vi "Cuboid Z test.vi"(1 "Cuboid 2":T1={"Vertices (x, y)"=[[0.0, 0.0], [0.0, 0.0], [0.0, 0.0], [0.0, 0.0]], "Zmin"=0.0, "Zmax"=0.0, "Centroid (x, y)"=[0.0, 0.0], "Radius"=0.0, "Edge normals (x, y)"=[[0.0, 0.0], [0.0, 0.0], [0.0, 0.0], [0.0, 0.0]], "Edge vectors (x, y)"=[[0.0, 0.0], [0.0, 0.0], [0.0, 0.0], [0.0, 0.0]]}, 2 "Cuboid 1":T1={"Vertices (x, y)"=[[0.0, 0.0], [0.0, 0.0], [0.0, 0.0], [0.0, 0.0]], "Zmin"=0.0, "Zmax"=0.0, "Centroid (x, y)"=[], "Radius"=0.0, "Edge normals (x, y)"=[[0.0, 0.0], [0.0, 0.0], [0.0, 0.0], [0.0, 0.0]], "Edge vectors (x, y)"=[[0.0, 0.0], [0.0, 0.0], [0.0, 0.0], [0.0, 0.0]]}) -> (0 "Possible collision":bool)   [LabVIEW 2013]
uses:
  Cuboid properties.ctl
panel:
  # "PN 30/08/2014"
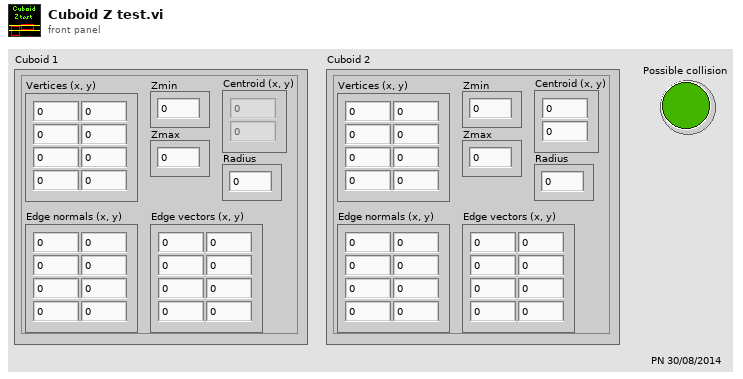
[diagram p1: front panel]
types:
  T1 = typedef "Cuboid properties.ctl" = cluster{"Vertices (x, y)":dbl[][], "Zmin":dbl, "Zmax":dbl, "Centroid (x, y)":dbl[], "Radius":dbl, "Edge normals (x, y)":dbl[][], "Edge vectors (x, y)":dbl[][]}
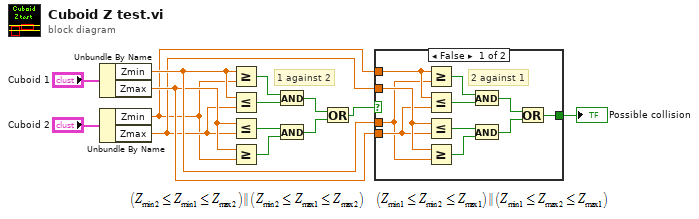
[diagram p0: block diagram]
diagram:
  # "1 against 2"
  n1 = Unbundle By Name("Cuboid 1") -> ("Zmin"=w4:dbl, "Zmax"=w3:dbl)
  n2 = Unbundle By Name("Cuboid 2") -> ("Zmin"=w1:dbl, "Zmax"=w2:dbl)
  n3 = Greater Or Equal?(x=w4, y=w1) -> (x >= y?=w10:bool)
  n4 = Less Or Equal?(x=w4, y=w2) -> (x <= y?=w9:bool)
  n5 = Less Or Equal?(x=w3, y=w2) -> (x <= y?=w8:bool)
  n6 = Greater Or Equal?(x=w3, y=w1) -> (x >= y?=w7:bool)
  n7 = And(x=w10, y=w9) -> (x .and. y?=w11:bool)
  n8 = And(x=w8, y=w7) -> (x .and. y?=w12:bool)
  n9 = Or(x=w11, y=w12) -> (x .or. y?=w6:bool)
  n10 = case shown="False" w6 {
    selector: w6 -> [_ w26]
    tunnel: [w19 w26] -> w5
    tunnel: w1 -> [w18 _]
    tunnel: w2 -> [w17 _]
    tunnel: w3 -> [w16 _]
    tunnel: w4 -> [w15 _]
    frame False {
      # "2 against 1"
      n11 = Greater Or Equal?(x=w18, y=w15) -> (x >= y?=w22:bool)
      n12 = Less Or Equal?(x=w18, y=w16) -> (x <= y?=w23:bool)
      n13 = Less Or Equal?(x=w17, y=w16) -> (x <= y?=w24:bool)
      n14 = Greater Or Equal?(x=w17, y=w15) -> (x >= y?=w25:bool)
      n15 = And(x=w22, y=w23) -> (x .and. y?=w21:bool)
      n16 = And(x=w24, y=w25) -> (x .and. y?=w20:bool)
      n17 = Or(x=w21, y=w20) -> (x .or. y?=w19:bool)
    }
    frame True {
      # "Already passed, no need to check 2 against 1"
    }
  }
  "Possible collision" <- w5
